vi "WorkerFactory.vi"(8 "error in (no error)":errorcluster, 11 "BuildWorker in":refnum<class "BuildWorker.lvclass">) -> (0 "error out":errorcluster, 1 "Port":u16, 2 "BuildWorkers":refnum<class "BuildWorker.lvclass">[](array[class]), 3 "BuildWorker out":refnum<class "BuildWorker.lvclass">, 4 "Show":bool)   [LabVIEW 2017, in "BuildWorker Controller.lvlib" / "BuildWorker.lvclass"]
uses:
  BuildWorker.lvclass
  BuildWorker.lvclass/BuildWorker.ctl
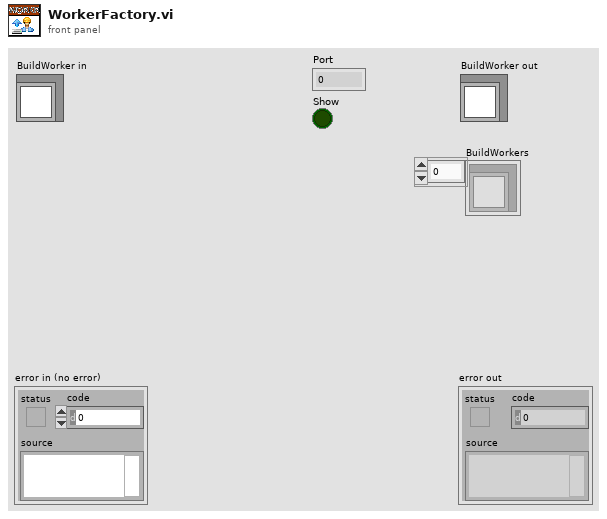
[diagram p1: front panel]
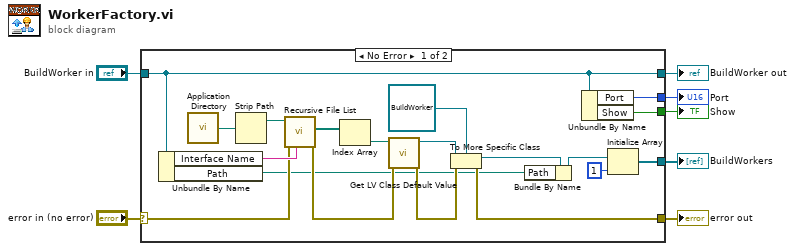
[diagram p0: block diagram]
diagram:
  n1 = case shown="No Error" "error in (no error)" {
    selector: "error in (no error)" -> [w25 w28]
    tunnel: [w19 w28] -> w6
    tunnel: [w16 w27] -> w4
    tunnel: "BuildWorker in" -> [w16 w27]
    tunnel: [w17 _] -> w3
    tunnel: [w12 _] -> w2
    tunnel: [w11 _] -> w1
    frame No Error {
      n2 = Unbundle By Name(w16) -> ("Interface Name"=w26:string, "Path"=w8:path)
      n3 = call <vilib>:"Application Directory.vi"() -> ("Application Directory"=w15:path)
      n4 = Strip Path(path=w15) -> (stripped path=w14:path)  [unwired: 1 out]
      n5 = call <vilib>:"Recursive File List.vi"("pattern"=w26, "error in (no error)"=w25, "Folder Path"=w14) -> ("error out"=w22:errorcluster, "All Files in Dir"=w24:path[])  [unwired: 4 in, 3 out]
      n6 = Index Array(array=w24) -> (element=w23:path)  [unwired: 1 in]
      n7 = call <vilib>:"Get LV Class Default Value.vi"("error in (no error)"=w22, "class path"=w23) -> ("error out"=w21:errorcluster, "object"=w20:refnum<class>)  [unwired: 8 in]
      n8 = To More Specific Class(target class=refnum<class "BuildWorker.lvclass"> refnum ("BuildWorker Controller.lvlib:BuildWorker.lvclass"), reference=w20, error in=w21) -> (specific class reference=w13:refnum<class "BuildWorker.lvclass">, error out=w19:errorcluster)
      n9 = Bundle By Name(cluster=w13, "Path"=w8) -> (w9:refnum<class "BuildWorker.lvclass">)
      n10 = Unbundle By Name(w16) -> ("Port"=w12:u16, "Show"=w11:bool)
      n11 = Initialize Array(w9, 1 ("dimension size")) -> (w17:refnum<class "BuildWorker.lvclass">[])
    }
    frame Error {
    }
  }
  "error out" <- w6
  "BuildWorker out" <- w4
  "BuildWorkers" <- w3
  "Port" <- w2
  "Show" <- w1
